vi "P1.vi"() -> ()   [LabVIEW 2021]
panel:
  out "Boolean":bool
  out "error out 2":errorcluster
  in  "String":string
  out "error out":errorcluster
  in  "Stop":bool
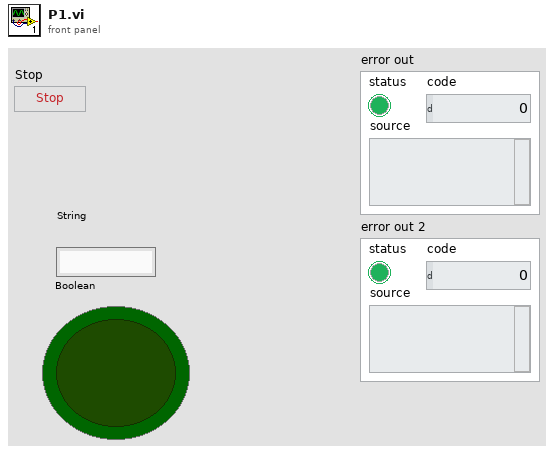
[diagram p1: front panel]
types:
  T1 = enum16{"Read", "Write", "ReadWrite", "BufferedRead", "BufferedReadWrite"}
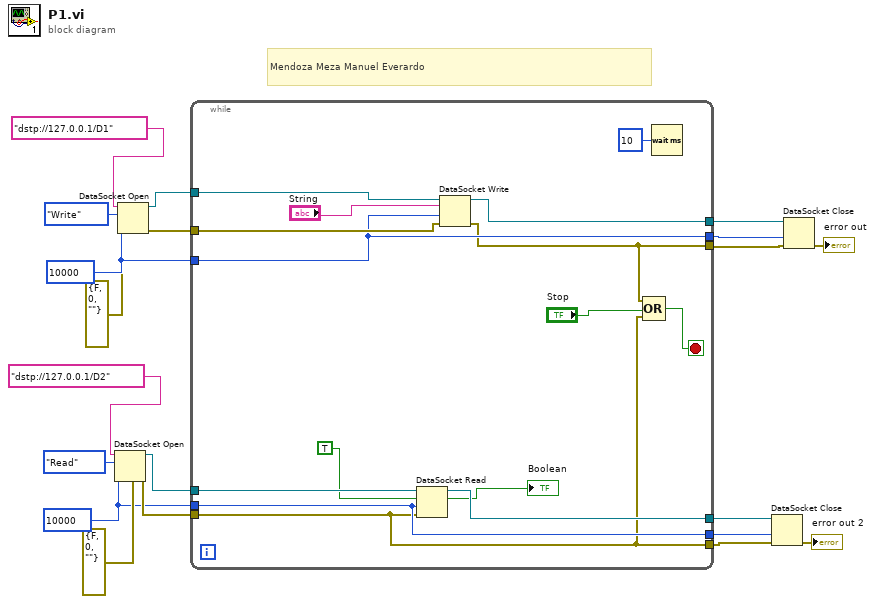
[diagram p0: block diagram]
diagram:
  w4 = 10000 ("ms timeout (10000)")
  w15 = 10000 ("ms timeout (10000)")
  # "Mendoza Meza Manuel Everardo"
  n1 = DataSocket Open(8:errorcluster {"status"=FALSE, "code"=0, "source"=""} ("error in (no error)"), 9:w4, 10:T1."Read" ("mode"), 11:"dstp://127.0.0.1/D2") -> (0:w6:errorcluster, 3:w7:refnum<k13>)
  n2 = DataSocket Open(8:errorcluster {"status"=FALSE, "code"=0, "source"=""} ("error in (no error)"), 9:w15, 10:T1."Write" ("mode"), 11:"dstp://127.0.0.1/D1") -> (0:w19:errorcluster, 3:w20:refnum<k13>)
  n3 = while {
    tunnel: w20 -> [w34]
    tunnel: w19 -> [w33]
    tunnel: [w28] -> w11
    tunnel: [w32] -> w18
    tunnel: w15 -> [w31]
    tunnel: [w31] -> w14
    tunnel: w7 -> [w26]
    tunnel: w6 -> [w21]
    tunnel: w4 -> [w25]
    tunnel: [w25] -> w3
    tunnel: [w21] -> w2
    tunnel: [w24] -> w1
    stop <- w29 stop-if-true
    n4 = DataSocket Read(8:w21, 9:w25, 10:TRUE, 11:w26) -> (2:→"Boolean":bool, 3:w24:refnum<k13>)  [unwired: 1 in, 5 out]
    n5 = DataSocket Write(8:w33, 9:w31, 10:"String", 11:w34) -> (0:w28:errorcluster, 3:w32:refnum<k13>)  [unwired: 1 out]
    n6 = Compound Arithmetic op=OR(w28, "Stop", w21) -> (w29:bool)
    n7 = Wait (ms)(milliseconds to wait=u32 10) -> ()  [unwired: 1 out]
  }
  n8 = DataSocket Close(8:w2, 9:w3, 11:w1) -> (0:→"error out 2":errorcluster)  [unwired: 1 out]
  n9 = DataSocket Close(8:w11, 9:w14, 11:w18) -> (0:→"error out":errorcluster)  [unwired: 1 out]
